vi "poly_search_vis_in_memory_exec_single.vi"(7 "app ref (open local)":refnum<vi>, 8 "error in (no error)":errorcluster, 9 "additional search items":T2={"+ in lvlibs"=TRUE, " + controls"=FALSE, " + self"=FALSE, "+ instances"=FALSE, "+ in llbs"=TRUE}, 10 "target exectuion state":T1(ring)) -> (0 "error out":errorcluster, 1 "vi paths":path[](array[path]), 2 "vi names":string[](array[string]), 5 "n of vis found":i32)   [LabVIEW 2015]
doc: "Check the execution state of all VIs in the current application (or in the app reference wired <- not tested). \n\nThe target execution states are\n - \"Run Top Level\" - Runnign vi\n - \"Running\" - Running sub vi\n - \"Idle\" - Loaded in memory but not running\n - \"Bad\" - Not executable\n\nYou can use additional search items to also specity whether to search for VIs in\n - lvlibs (T)\n - llbs (T)\n - .ctl files (F)\n - reetnant instances (F)\n - this vi (F)"
uses:
  misc_tools/SearchItems.ctl
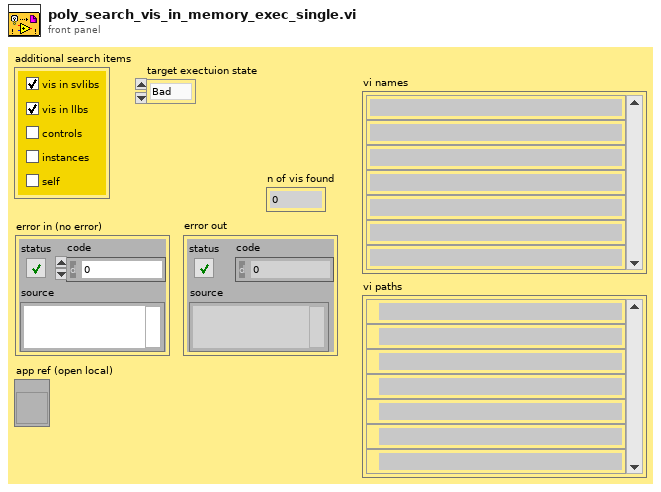
[diagram p1: front panel]
types:
  T1 = enum32{"Bad", "Idle", "Run top level", "Running"}
  T2 = typedef "SearchItems.ctl" = cluster{"+ in lvlibs":bool, " + controls":bool, " + self":bool, "+ instances":bool, "+ in llbs":bool}
  T3 = enum32{"Bad", "Idle", "Run top level", "Running"}[]
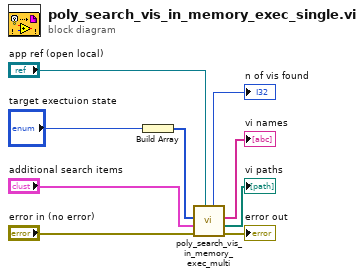
[diagram p0: block diagram]
diagram:
  n1 = Build Array("target exectuion state") -> (w8:T3)
  n2 = call "poly_search_vis_in_memory_exec_multi.vi"("app ref (open local)"="app ref (open local)", "error in (no error)"="error in (no error)", "additional search items"="additional search items", "tagert exectution states"=w8) -> ("error out"=→"error out":errorcluster, "vi paths"=→"vi paths":path[], "vi names"=→"vi names":string[], "n of vis found"=→"n of vis found":i32)  [unwired: 4 in]
